vi "Destructor.vi"(8 "error in (no error)":errorcluster, 11 "VIActivation in":refnum<class "VIActivation.lvclass">) -> (0 "error out":errorcluster)   [LabVIEW 2021, in "VIActivation.lvlib" / "VIActivation.lvclass"]
uses:
  VIActivation.lvclass
  VIActivation.lvclass/VIActivation.ctl
  8a170fa0-6211-4169-a003-11f440d964db.vi
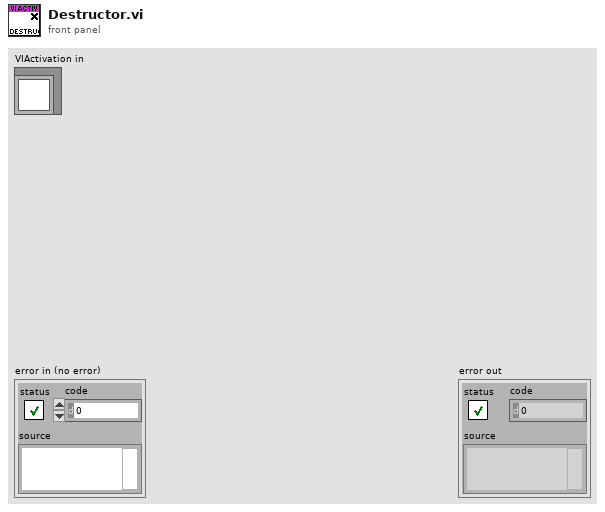
[diagram p1: front panel]
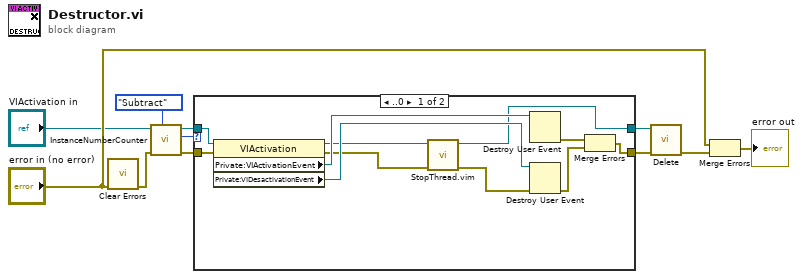
[diagram p0: block diagram]
diagram:
  n1 = call <vilib>:"Clear Errors.vi"("error in (no error)"="error in (no error)") -> ("error out"=w9:errorcluster)  [unwired: 5 in, 1 out]
  n2 = call "InstanceNumberCounter.vi"("Action"=enum16{"Get", "Add", "Subtract"}."Subtract", "error in (no error)"=w9, "VI Activation in"="VIActivation in") -> ("error out"=w5:errorcluster, "InstanceNumber out"=w6:i32, "VI Activation out"=w4:refnum<class "VIActivation.lvclass">)  [unwired: 6 in]
  n3 = case shown="..0" w6 {
    tunnel: w5 -> [w22 w23]
    tunnel: w4 -> [w18 w24]
    tunnel: [w19 w23] -> w3
    tunnel: [w14 w24] -> w1
    frame ..0 {
      n4 = property class="VIActivation"(reference=w18, error in=w22) -> (reference out=w15:refnum<class "VIActivation.lvclass">, error out=w13:errorcluster, "Private:VIActivationEvent"=w17:refnum<user-event>, "Private:VIDesactivationEvent"=w16:refnum<user-event>)
      n5 = call "StopThread.vim"("error in (no error)"=w13, "ByRefClass in"=w15) -> ("error out"=w12:errorcluster, "ByRefClass out"=w14:refnum<class "VIActivation.lvclass">)  [unwired: 8 in]
      n6 = Destroy User Event(user event=w17) -> (error out=w21:errorcluster)  [unwired: 1 in]
      n7 = Destroy User Event(user event=w16, error in=w12) -> (error out=w20:errorcluster)
      n8 = Merge Errors(w21, w20) -> (w19:errorcluster)
    }
    frame Default {
    }
  }
  n9 = call-dynamic "Delete.vi"("error in (no error)"=w3, "ByRefClass in"=w1) -> ("error out"=w2:errorcluster)  [unwired: 8 in, 1 out]
  n10 = Merge Errors("error in (no error)", w2) -> (→"error out":errorcluster)
